vi "Erase Message.vi"(8 "error in (no error)":errorcluster, 11 "SPARC4_GUI in":refnum<class "SPARC4_GEI.lvclass">) -> (0 "error out":errorcluster, 3 "SPARC4_GUI out":refnum<class "SPARC4_GEI.lvclass">)   [LabVIEW 2018, in "SPARC4_GEI.lvclass"]
uses:
  SPARC4_GEI.lvclass
  SPARC4_GEI.lvclass/SPARC4_GEI.ctl
  Channel GUI/Channel GEI.lvclass
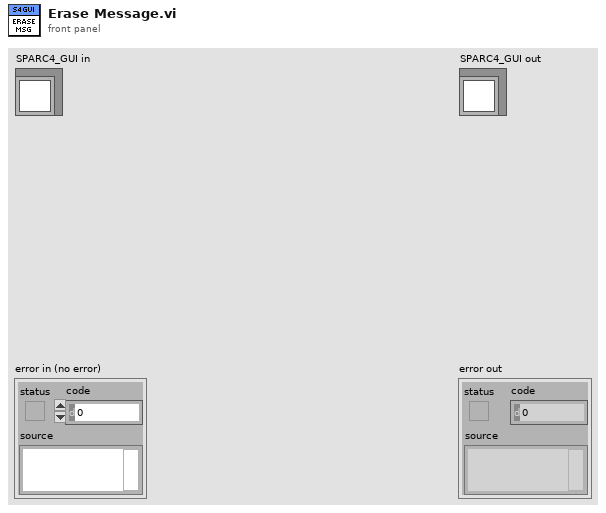
[diagram p1: front panel]
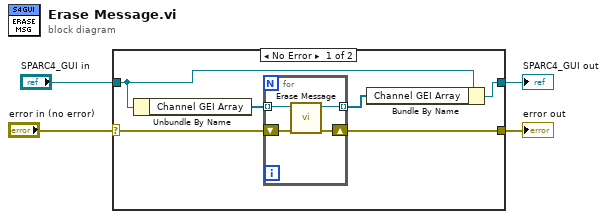
[diagram p0: block diagram]
diagram:
  n1 = case shown="No Error" "error in (no error)" {
    selector: "error in (no error)" -> [w7 w16]
    tunnel: [w8 w16] -> w3
    tunnel: [w9 w15] -> w1
    tunnel: "SPARC4_GUI in" -> [w10 w15]
    frame No Error {
      n2 = Unbundle By Name(w10) -> ("Channel GEI Array"=w6:refnum<class "Channel GEI.lvclass">[])
      n3 = for {
        tunnel: w6 -> [w12] mode=indexing
        tunnel: [w11] -> w5 mode=indexing
        shift-right: [w14] -> w8
        shift-left: w7 -> [w13]
        n4 = call "Erase Message.vi"("error in (no error)"=w13, "Channel GUI in"=w12) -> ("error out"=w14:errorcluster, "Channel GUI out"=w11:refnum<class "Channel GEI.lvclass">)  [unwired: 8 in]
      }
      n5 = Bundle By Name(cluster=w10, "Channel GEI Array"=w5) -> (w9:refnum<class "SPARC4_GEI.lvclass">)
    }
    frame Error {
    }
  }
  "error out" <- w3
  "SPARC4_GUI out" <- w1
